vi "Set Port Number.vi"(8 "error in":errorcluster, 10 "port number":u16, 11 "port ref":T1 format="%.0x") -> (0 "error out":errorcluster, 3 "port ref out":T1 format="%.0x")   [LabVIEW 2020, in "AIM ARINC 429 Scripting.lvlib"]
uses:
  AIM ARINC 429 Scripting.lvlib
  <vilib>/NI VeriStand/Custom Device API/Custom Device Item Ref.ctl
  Constants.vi
  <vilib>/NI VeriStand/Custom Device API/Set Item Property (U16).vi
  <vilib>/NI VeriStand/Custom Device API/Custom Device API.lvlib
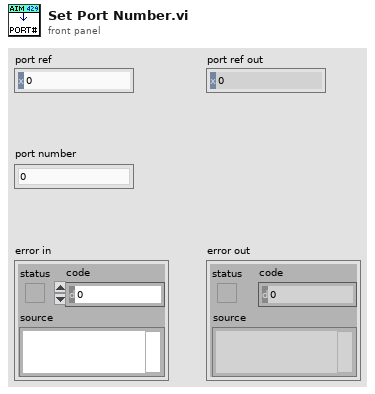
[diagram p1: front panel]
types:
  T1 = typedef "Custom Device API.lvlib/Custom Device Item Ref.ctl" = u64
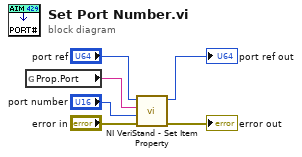
[diagram p0: block diagram]
diagram:
  n1 = global read "Constants.vi" "Prop.Port"() -> (w2:string)
  n2 = call-poly <vilib>:"NI VeriStand - Set Item Property.vi"("error in (no error)"="error in", "Value"="port number", "Property Name"=w2, "Item Ref in"="port ref") -> ("error out"=→"error out":errorcluster, "Item Ref out"=→"port ref out":T1)  [unwired: 5 in, 1 out]
